vi "Sequence Global.vi"(4 "String Indicator":refnum<vi>, 6 "Table Ref In":refnum<vi>, 8 "Action":T7, 10 "New Seq Index":i32, 11 "Sequence List In":T1[](array[typedef])) -> (1 "Current Index":i32, 2 "Current Sequence":T1, 3 "Sequence List Out":T1[](array[typedef]))   [LabVIEW 2015]
uses:
  Sequence Global Action.ctl
  Sequence File IO/Single Test Sequence.ctl
  Test Sequence Action.ctl
  Valve Action Enum.ctl
  Valve Name Enum.ctl
  Sequence File IO/Test Sequence Trigger.ctl
  Sensors/Sensor Enum.ctl
panel:
  out "Table Ref":refnum<vi>
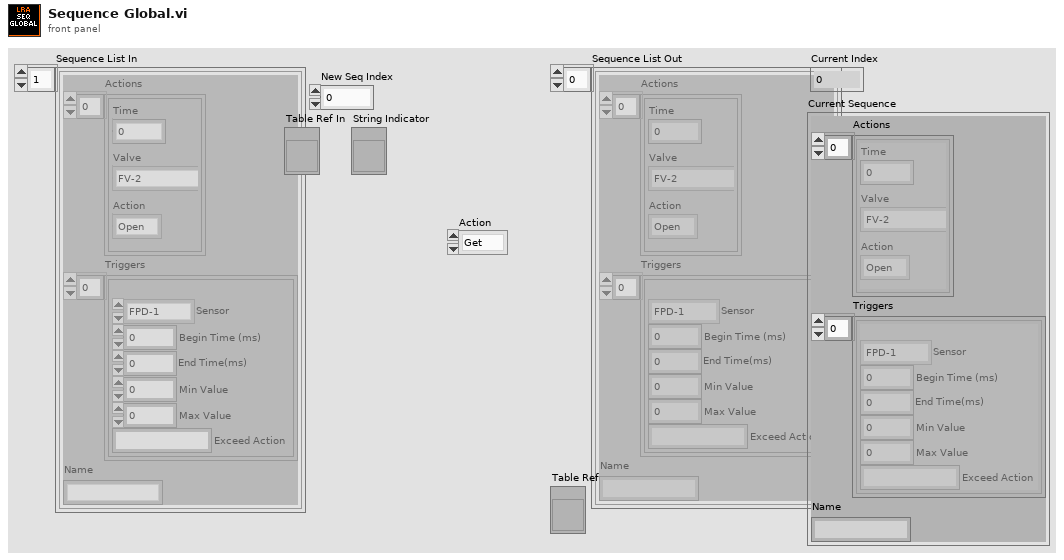
[diagram p1: front panel]
types:
  T1 = typedef "Single Test Sequence.ctl" = cluster{"Actions":T2[], "Triggers":T5[], "Name":string}
  T2 = typedef "Test Sequence Action.ctl" = cluster{"Time":i32, "Action":T3, "Valve":T4}
  T3 = typedef "Valve Action Enum.ctl" = enum16{"Open", "Close"}
  T4 = typedef "Valve Name Enum.ctl" = enum16{"FV-2", "FV-3", "FV-4", "OV-2", "OV-3", "OV-4", "COMP"}
  T5 = typedef "Test Sequence Trigger.ctl" = cluster{"Sensor":T6, "Begin Time (ms)":u32, "End Time(ms)":u32, "Min Value":dbl, "Max Value":dbl, "Exceed Action":string}
  T6 = typedef "Sensor Enum.ctl" = enum16{"FPD-1", "FPD-2", "FPD-3", "OPD-1", "OPD-2", "OPD-3", "AP-1", "VBAT", "VCOMP", "ICOMP", "TD10"}
  T7 = typedef "Sequence Global Action.ctl" = enum16{"Get", "Set List", "Set Current"}
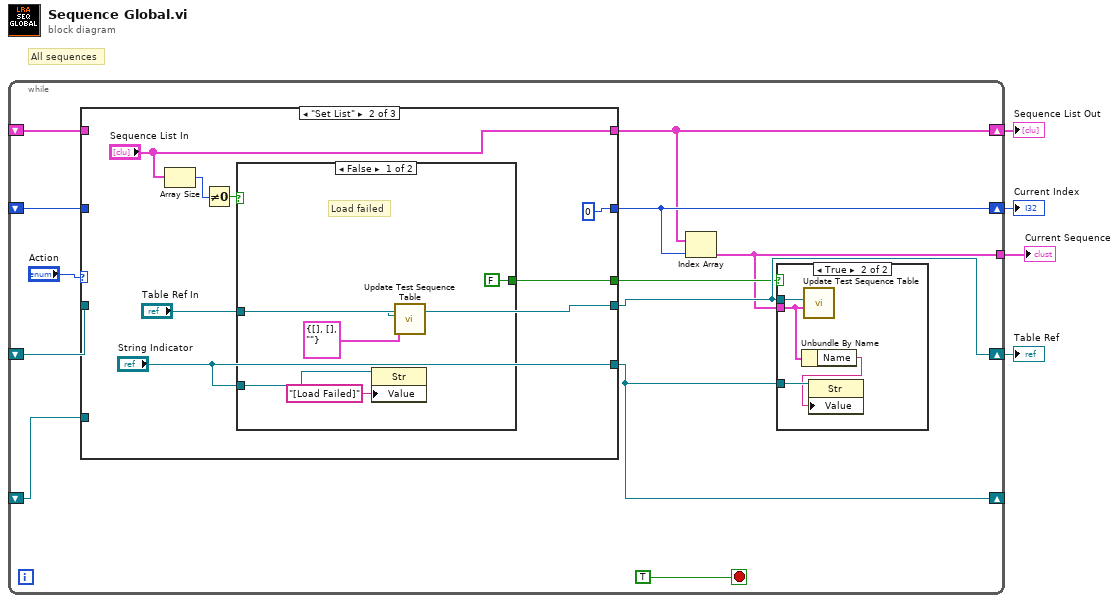
[diagram p0: block diagram]
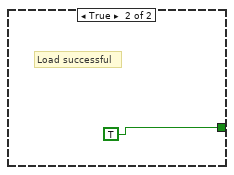
[diagram p4: hidden frame]
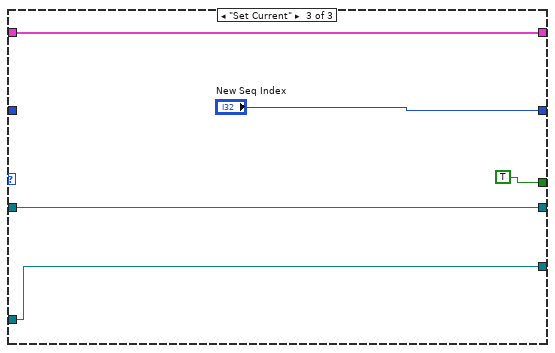
[diagram p5: hidden frame]
diagram:
  # "All sequences"
  n1 = while {
    shift-right: [w5] -> w4
    shift-left: _ -> [w14]
    shift-right: [w12] -> w3
    shift-left: _ -> [w13]
    tunnel: [w8] -> w2
    shift-right: [w10] -> w1
    shift-left: _ -> [w11]
    shift-right: [w7] -> _
    shift-left: _ -> [w6]
    stop <- TRUE stop-if-true
    n2 = case shown="\"Set List\"" "Action" {
      tunnel: w14 -> [w24 _ w42]
      tunnel: [w24 "Sequence List In" w42] -> w5
      tunnel: [w23 0 "New Seq Index"] -> w12
      tunnel: w13 -> [w23 _ _]
      tunnel: w11 -> [w22 _ w40]
      tunnel: [w22 "Table Ref In" w40] -> w10
      tunnel: [_ w27 TRUE] -> w9
      tunnel: [w21 "String Indicator" w38] -> w7
      tunnel: w6 -> [w21 _ w38]
      frame "Get" {
      }
      frame "Set List" {
        n3 = Array Size(array="Sequence List In") -> (size(s)=w29:i32)
        n4 = Not Equal To 0?(x=w29) -> (x != 0?=w28:bool)
        n5 = case shown="False" w28 {
          tunnel: [FALSE TRUE] -> w27
          tunnel: "String Indicator" -> [w36 _]
          tunnel: "Table Ref In" -> [w33 _]
          frame False {
            # "Load failed"
            n6 = property class="Str"(reference=w36, "Value"="[Load Failed]") -> ()  [unwired: 1 in, 2 out]
            n7 = call "Update Test Sequence Table.vi"("Test Sequence"=T1 {"Actions"=[], "Triggers"=[], "Name"=""}, "reference"=w33) -> ()  [unwired: 10 in]
          }
          frame True {
            # "Load successful"
          }
        }
      }
      frame "Set Current" {
      }
    }
    n8 = Index Array(array=w5, index=w12) -> (element=w8:T1)
    n9 = case shown="True" w9 {
      tunnel: w8 -> [_ w19]
      tunnel: w10 -> [_ w20]
      tunnel: w7 -> [_ w18]
      frame False {
      }
      frame True {
        n10 = Unbundle By Name(w19) -> ("Name"=w17:string)
        n11 = call "Update Test Sequence Table.vi"("Test Sequence"=w19, "reference"=w20) -> ()  [unwired: 10 in]
        n12 = property class="Str"(reference=w18, "Value"=w17) -> ()  [unwired: 1 in, 2 out]
      }
    }
  }
  "Sequence List Out" <- w4
  "Current Index" <- w3
  "Current Sequence" <- w2
  "Table Ref" <- w1
